vi "Add ROI Offset RectFilter.vi"(4 "Region of Interest":i32[](array[numeric])=[-1, -1, 32000, 32000], 5 "RectFilter In":T1 {"Rotation" format="%.2f"; "Left" scale=0.0..1024.0; "Right" scale=0.0..1024.0}) -> (2 "RectFilter Out":T1 {"Rotation" format="%.2f"; "Left" scale=0.0..1024.0; "Right" scale=0.0..1024.0})   [LabVIEW 2013]
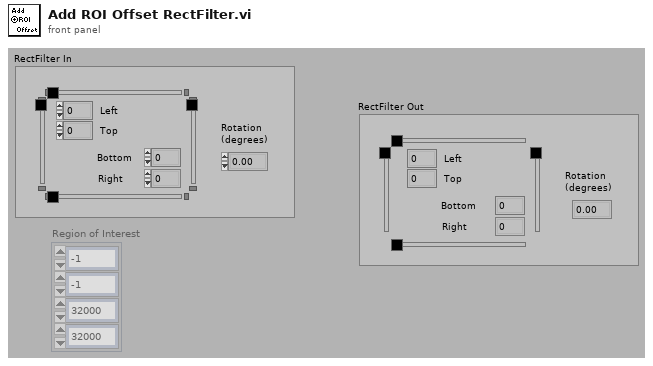
[diagram p1: front panel]
types:
  T1 = typedef "IMAQ Rectangle" = cluster{"Left":i32, "Top":i32, "Right":i32, "Bottom":i32, "Rotation":dbl}
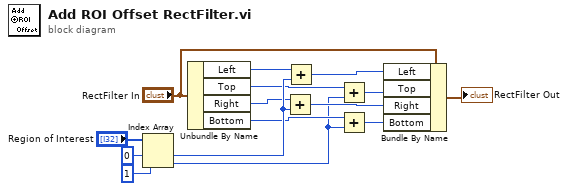
[diagram p0: block diagram]
diagram:
  n1 = Index Array(array="Region of Interest", index #1=0 ("index"), index #2=1 ("index")) -> (element #1=w10:i32, element #2=w2:i32)
  n2 = Unbundle By Name("RectFilter In") -> ("Left"=w9:i32, "Top"=w6:i32, "Right"=w8:i32, "Bottom"=w4:i32)
  n3 = Add(x=w8, y=w10) -> (x+y=w5:i32)
  n4 = Add(x=w9, y=w10) -> (x+y=w7:i32)
  n5 = Add(x=w6, y=w2) -> (x+y=w1:i32)
  n6 = Add(x=w4, y=w2) -> (x+y=w3:i32)
  n7 = Bundle By Name(cluster="RectFilter In", "Left"=w7, "Top"=w1, "Right"=w5, "Bottom"=w3) -> (→"RectFilter Out":T1)
